vi "Dialog.vi"(5 "Window Position (Center in Top Level)":refnum<class "Window Position.lvclass">, 6 "Behavior (Modal)":T1=enum."Modal", 7 "Autoshow? (T)":bool=TRUE, 8 "Error In":errorcluster, 10 "Default Title":string) -> (0 "Error Out":errorcluster, 3 "Dialog out":refnum<class "Dialog.lvclass">)   [LabVIEW 2023, in "Panel Actor.lvlib" / "Panel.lvlib" / "Dialog.lvclass"]
doc: "Creates a new dialog. A dialog is just like a normal window except it's FP will be set to modal or Floating before it's shown.\n\nA Dialog is repositioned every time it is shown.\n\n<B>Default Title:</B> Sets the default title for the window.\n<B>Autoshow?</B> If Autoshow? is TRUE, then the Window will be displayed on initialization. If it is FALSE, then the Show method must be called manually.\n<B>Window Position:</B> Window Position object to control window position behavior.\n<B>Behavior (Modal):</B> Sets the window behavior for the dialog.\n<B>Error In:</B> Describes error conditions that occur before this node runs.\n\n<B>Window Out:</B> New Window object.\n<B>Error Out:</B> Contains error information.\n----\nPlease see the following web address for additional documentation and tutorial information:\nhttp://www.mooregoodideas.com/mgi-panel-manager/\n\nAuthor: Derek Trepanier\n\nCopyright (c) 2018, Moore Good Ideas, Inc.\n\nAll rights reserved.\n\nRedistribution and use in source and binary forms, with or without modification, are permitted provided that the following conditions are met:\n\n * Redistributions of source code must retain the above copyright notice, this list of conditions and the following disclaimer.\n * Redistributions in binary form must reproduce the above copyright notice, this list of conditions and the following disclaimer in the documentation and/or other materials provided with the distribution.\n * Neither the name of Moore Good Ideas, Inc. nor the names of its contributors may be used to endorse or promote products derived from this software without specific prior written permission.\n\nTHIS SOFTWARE IS PROVIDED BY THE COPYRIGHT HOLDERS AND CONTRIBUTORS \"AS IS\" AND ANY EXPRESS OR IMPLIED WARRANTIES, INCLUDING, BUT NOT LIMITED TO, THE IMPLIED WARRANTIES OF MERCHANTABILITY AND FITNESS FOR A PARTICULAR PURPOSE ARE DISCLAIMED. IN NO EVENT SHALL THE COPYRIGHT OWNER OR CONTRIBUTORS BE LIABLE FOR ANY DIRECT, INDIRECT, INCIDENTAL, SPECIAL, EXEMPLARY, OR CONSEQUENTIAL DAMAGES (INCLUDING, BUT NOT LIMITED TO, PROCUREMENT OF SUBSTITUTE GOODS OR SERVICES; LOSS OF USE, DATA, OR PROFITS; OR BUSINESS INTERRUPTION) HOWEVER CAUSED AND ON ANY THEORY OF LIABILITY, WHETHER IN CONTRACT, STRICT LIABILITY, OR TORT (INCLUDING NEGLIGENCE OR OTHERWISE) ARISING IN ANY WAY OUT OF THE USE OF THIS SOFTWARE, EVEN IF ADVISED OF THE POSSIBILITY OF SUCH DAMAGE."
uses:
  Dialog.lvclass
  Behavior.ctl
  Window Position/Window Position.lvclass
  Dialog.lvclass/Dialog.ctl
  Window Position/Reference Position/Ref Top Level/Ref Top Level.lvclass
  Window.lvclass
  C:/Users/Public/Documents/Development/Engine/Panel Manager/Panel/Window Position/Reference Position/Reference Position.lvclass
  C:/Users/Public/Documents/Development/Engine/Panel Manager/Panel/Window Position/Window Position.lvclass
  C:/Users/Public/Documents/Development/Engine/Panel Manager/Panel/Window Position/Reference Position/Ref Top Level/Ref Top Level.lvclass
  C:/Users/Public/Documents/Development/Engine/Panel Manager/Panel/Panel/Window/Window.lvclass
  C:/Users/Public/Documents/Development/Engine/Panel Manager/Panel/Panel/Panel.lvclass
  C:/Users/Public/Documents/Development/Engine/Panel Manager/Panel/Panel/Window/Dialog/Dialog.lvclass
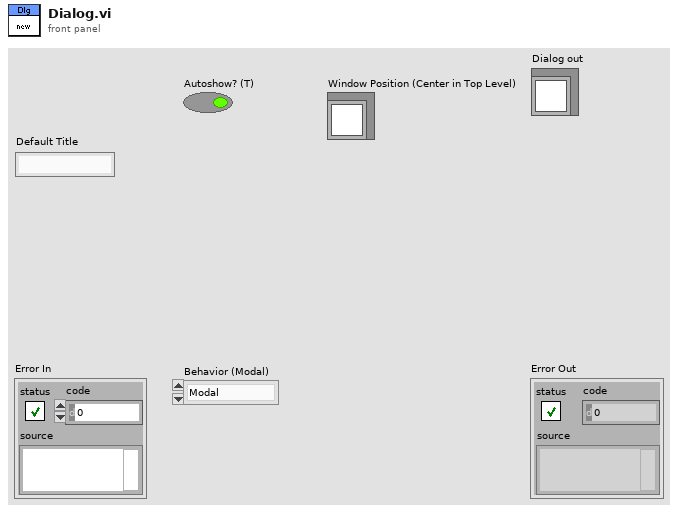
[diagram p1: front panel]
types:
  T1 = typedef "Panel Actor.lvlib/Panel.lvlib/Dialog.lvclass/Behavior.ctl" = enum32{"Floating", "Floating/Auto-Hide", "Modal"}
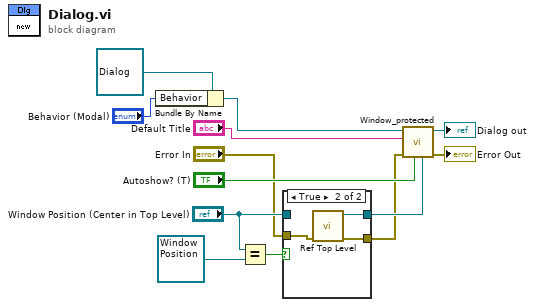
[diagram p0: block diagram]
diagram:
  n1 = Bundle By Name(cluster=refnum<class "Dialog.lvclass"> refnum ("Dialog in"), "Behavior"="Behavior (Modal)") -> (w8:refnum<class "Dialog.lvclass">)
  n2 = Equal?(x="Window Position (Center in Top Level)", y=refnum<class "Window Position.lvclass"> refnum ("Panel.lvlib:Window Position.lvclass")) -> (x = y?=w5:bool)
  n3 = case shown="True" w5 {
    tunnel: [w15 w18] -> w4
    tunnel: "Window Position (Center in Top Level)" -> [w15 _]
    tunnel: "Error In" -> [w14 w17]
    tunnel: [w14 w16] -> w1
    frame False {
    }
    frame True {
      n4 = call "Ref Top Level.vi"("Error In"=w17) -> ("Error Out"=w16:errorcluster, "Ref Top Level out"=w18:refnum<class "Ref Top Level.lvclass">)  [unwired: 9 in]
    }
  }
  n5 = call "Window_protected.vi"("Window Position"=w4, "Autoshow?"="Autoshow? (T)", "error in (no error)"=w1, "Default Title"="Default Title", "Window in"=w8) -> ("error out"=→"Error Out":errorcluster, "Window in"=→"Dialog out":refnum<class "Dialog.lvclass">)  [unwired: 5 in]
